vi "Increment Patch.vi"(8 "error in (no error)":errorcluster, 10 "selected path":path) -> (0 "error out":errorcluster, 2 "VI Package Build Spec Data":T1)   [LabVIEW 2019, in "VIPM.lvclass"]
uses:
  VIPM.lvclass
  <vilib>/JKI/VIPM API/command-line/support/VI Package Build Spec Data Cluster_vipm_api.ctl
  <vilib>/JKI/VIPM API/command-line/support/Version Info Cluster_vipm_api.ctl
  <vilib>/JKI/VIPM API/VIPM API_vipm_api.lvlib
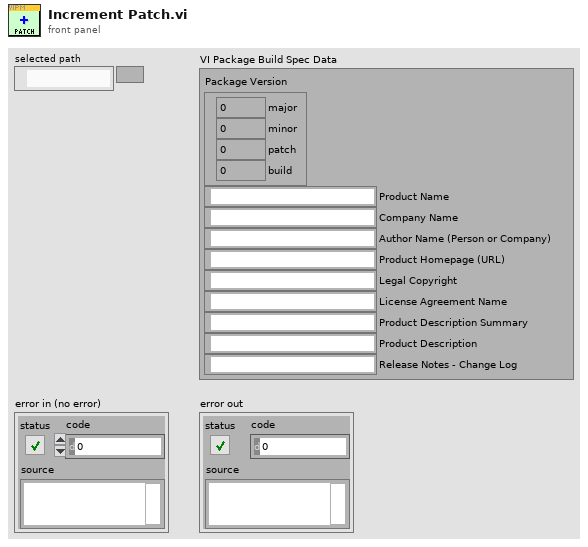
[diagram p1: front panel]
types:
  T1 = typedef "VIPM API_vipm_api.lvlib/VI Package Build Spec Data Cluster_vipm_api.ctl" = cluster{"Package Version":T2, "Product Name":string, "Company Name":string, "Author Name (Person or Company)":string, "Product Homepage (URL)":string, "Legal Copyright":string, "License Agreement Name":string, "Product Description Summary":string, "Product Description":string, "Release Notes - Change Log":string}
  T2 = typedef "VIPM API_vipm_api.lvlib/Version Info Cluster_vipm_api.ctl" = cluster{"major":u32, "minor":u32, "patch":u32, "build":u32}
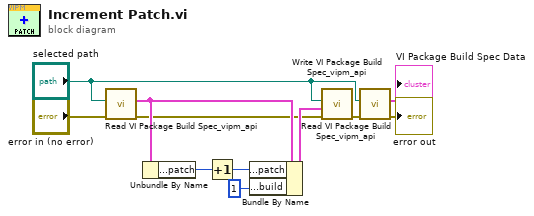
[diagram p0: block diagram]
diagram:
  n1 = call <vilib>:"Read VI Package Build Spec_vipm_api.vi"("error in (no error)"="error in (no error)", "Path to VIPB File"="selected path") -> ("error out"=w2:errorcluster, "VI Package Build Spec Data"=w3:T1)  [unwired: 8 in]
  n2 = Unbundle By Name(w3) -> ("Package Version.patch"=w11:u32)
  n3 = Increment(x=w11) -> (x+1=w4:u32)
  n4 = Bundle By Name(cluster=w3, "Package Version.patch"=w4, "Package Version.build"=u32 1) -> (w5:T1)
  n5 = call <vilib>:"Write VI Package Build Spec_vipm_api.vi"("error in (no error)"=w2, "VI Package Build Spec Data"=w5, "Path to VIPB File"="selected path") -> ("error out"=w6:errorcluster)  [unwired: 8 in]
  n6 = call <vilib>:"Read VI Package Build Spec_vipm_api.vi"("error in (no error)"=w6, "Path to VIPB File"="selected path") -> ("error out"=→"error out":errorcluster, "VI Package Build Spec Data"=→"VI Package Build Spec Data":T1)  [unwired: 8 in]
